vi "KGN Get MFC Flow.vi"(8 "Fehler (Eingang, kein Fehler)":errorcluster, 9 "Info Cluster":T1, 10 "VISA-Ressourcenname":refnum<visa-resource-name>, 11 "device (Eingang)":u32) -> (0 "Fehler (Ausgang)":errorcluster, 1 "Info Cluster out":T1, 2 "VISA-Ressourcenname out":refnum<visa-resource-name>, 3 "dup device (Ausgang)":u32, 4 "MFC Flows (Ausgang)":T2(array[cluster]), 6 "Kommandos gesendet":string)   [LabVIEW 2020, in "Linearisierung v2.lvlib" / "Gasteiler.lvlib" / "HovaCAL_Interface.lvlib" / "KGN.lvlib" / "KGN GUI Get.lvlib"]
uses:
  KGN GUI Get.lvlib
  Controls/Info Cluster.ctl
  get/get.lvlib
  Controls/Controls.lvlib
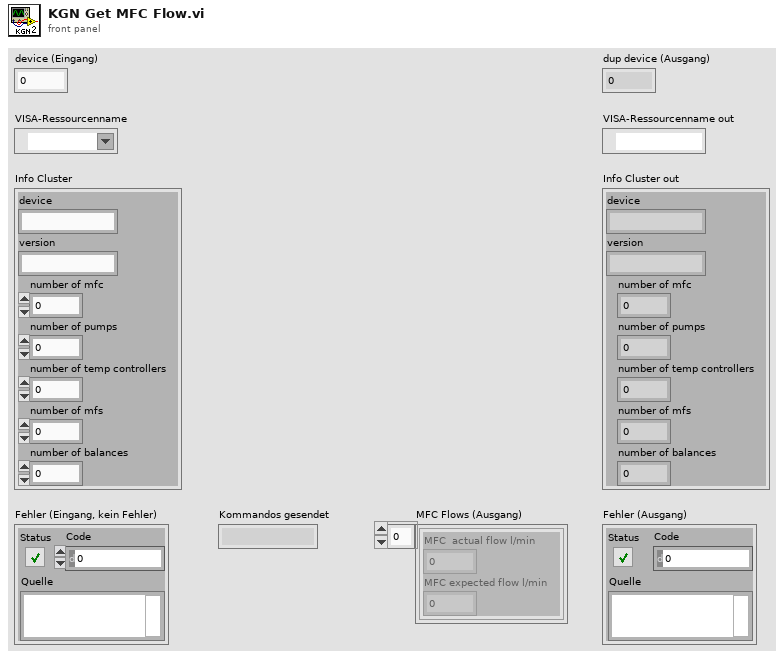
[diagram p1: front panel]
types:
  T1 = typedef "Linearisierung v2.lvlib/Gasteiler.lvlib/HovaCAL_Interface.lvlib/Controls.lvlib/Info Cluster.ctl" = cluster{"device":string, "version":string, "number of mfc":i32, "number of pumps":i32, "number of temp controllers":i32, "number of mfs":i32, "number of balances":i32}
  T2 = cluster{"MFC  actual flow l/min":dbl, "MFC expected flow l/min":dbl}[]
  T3 = cluster{"MFC  actual flow l/min":dbl, "MFC expected flow l/min":dbl}
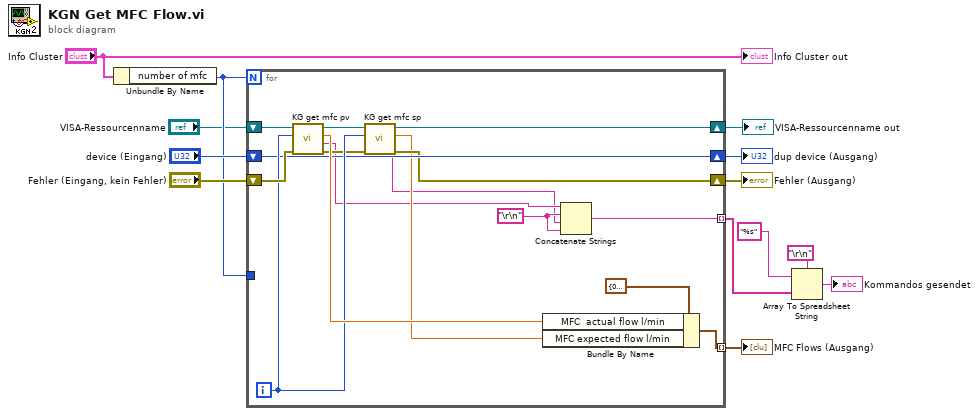
[diagram p0: block diagram]
diagram:
  n1 = Unbundle By Name("Info Cluster") -> ("number of mfc"=w8:i32)
  n2 = for {
    N: w8 -> [_]
    tunnel: w8 -> [_]
    tunnel: [w29] -> w5 mode=indexing
    shift-right: [w20] -> w12
    shift-left: "Fehler (Eingang, kein Fehler)" -> [w27]
    shift-right: [w25] -> w13
    shift-left: "device (Eingang)" -> [w25]
    shift-right: [w21] -> w6
    shift-left: "VISA-Ressourcenname" -> [w24]
    tunnel: [w14] -> w2 mode=indexing
    i -> [w26]
    w17 = "\r\n"
    n3 = call "KG get mfc pv.vi"("Fehler (Eingang, kein Fehler)"=w27, "mfc"=w26, "VISA-Ressourcenname"=w24) -> ("Fehler (Ausgang)"=w22:errorcluster, "Kommando gesendet"=w16:string, "flow"=w28:dbl, "VISA-Ressourcenname (Ausgang)"=w23:refnum<visa-resource-name>)  [unwired: 5 in]
    n4 = call "KG get mfc sp.vi"("Fehler (Eingang, kein Fehler)"=w22, "mfc"=w26, "VISA-Ressourcenname"=w23) -> ("Fehler (Ausgang)"=w20:errorcluster, "Kommando gesendet"=w15:string, "flow"=w18:dbl, "VISA-Ressourcenname (Ausgang)"=w21:refnum<visa-resource-name>)  [unwired: 5 in]
    n5 = Bundle By Name(cluster=T3 {"MFC  actual flow l/min"=0.0, "MFC expected flow l/min"=0.0} ("Actual Values Cluster"), "MFC  actual flow l/min"=w28, "MFC expected flow l/min"=w18) -> (w29:T3)
    n6 = Concatenate Strings(w16, w17, w15, w17) -> (w14:string)
  }
  "MFC Flows (Ausgang)" <- w5
  "dup device (Ausgang)" <- w13
  "Fehler (Ausgang)" <- w12
  "VISA-Ressourcenname out" <- w6
  n7 = Array To Spreadsheet String(delimiter (Tab)="\r\n", array=w2, 3:"%s" ("Format-String")) -> (spreadsheet string=→"Kommandos gesendet":string)
  "Info Cluster out" <- "Info Cluster"
